vi "BK Precision 5490C Series Acquire Single.vi"(6 "Auto Range (T: Enable)":bool=TRUE, 7 "Open?":bool=TRUE, 8 "error in":errorcluster, 9 "Manual Range (1)":dbl=1.0, 10 "Measurement Function (0: Voltage DC)":i32(ring) items=["Voltage DC", "Voltage DC Ratio", "Voltage AC", "Current DC", "Current AC", "Resistance 2-Wire", "Resistance 4-Wire", "Frequency", "Period", "Capacitance", "Continuity", "Diode", "Temperature"], 11 "VISA resource name":refnum<visa-resource-name>="USB0::0x3121::0x5000::556K20102::INSTR") -> (0 "error out":errorcluster, 3 "Measurement":dbl)   [LabVIEW 2018]
doc: "This example shows how to acquire a single triggered measurement."
uses:
  <instrlib>/BK Precision 5490C Series/Public/Data/Read (Single Point).vi
  <instrlib>/BK Precision 5490C Series/BK Precision 5490C Series.lvlib
panel:
  # "(c) 2020 B&K Precision Corporation.  ALL RIGHTS RESERVED."
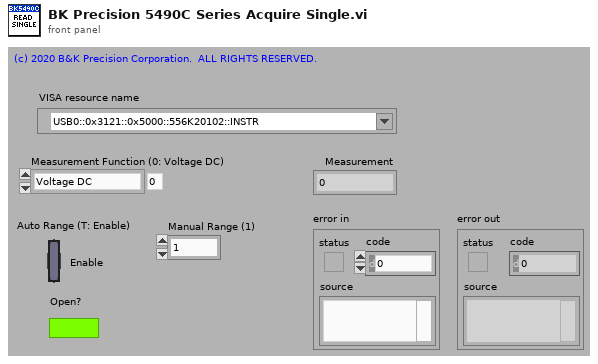
[diagram p1: front panel]
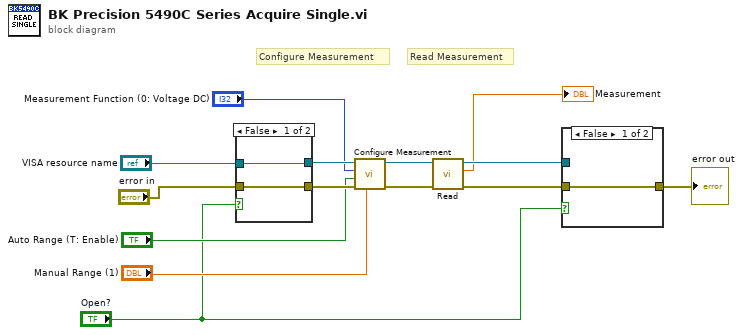
[diagram p0: block diagram]
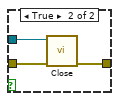
[diagram p2: hidden frame]
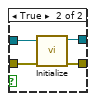
[diagram p3: hidden frame]
diagram:
  # "Read Measurement"
  # "Configure Measurement"
  n1 = case shown="False" "Open?" {
    tunnel: [w16 w20] -> w14
    tunnel: [w15 w19] -> w13
    tunnel: "VISA resource name" -> [w16 w18]
    tunnel: "error in" -> [w15 w17]
    frame False {
    }
    frame True {
      n2 = call <instrlib>:"Initialize.vi"("error in (no error)"=w17, "VISA resource name"=w18) -> ("error out"=w19:errorcluster, "VISA resource name out"=w20:refnum<visa-resource-name>)  [unwired: 3 in, 5 out]
    }
  }
  n3 = call <instrlib>:"Configure Measurement.vi"("Manual Range (1)"="Manual Range (1)", "error in (no error)"=w13, "Auto Range (T: Enable)"="Auto Range (T: Enable)", "Measurement Function (0: Voltage DC)"="Measurement Function (0: Voltage DC)", "VISA resource name"=w14) -> ("error out"=w9:errorcluster, "VISA resource name out"=w10:refnum<visa-resource-name>)  [unwired: 1 in, 4 out]
  n4 = call-poly <instrlib>:"Read.vi"("error in (no error)"=w9, "VISA resource name"=w10) -> ("error out"=w12:errorcluster, "Measurement"=→"Measurement":dbl, "VISA resource name out"=w11:refnum<visa-resource-name>)  [unwired: 7 out]
  n5 = case shown="False" "Open?" {
    tunnel: w12 -> [w21 w24]
    tunnel: w11 -> [_ w23]
    tunnel: [w21 w22] -> w3
    frame False {
    }
    frame True {
      n6 = call <instrlib>:"Close.vi"("error in (no error)"=w24, "VISA resource name"=w23) -> ("error out"=w22:errorcluster)  [unwired: 9 out]
    }
  }
  "error out" <- w3
